vi "Write useUTC.vi"(8 "error in (no error)":errorcluster, 10 "useUTC":bool, 11 "Layout in":refnum<class "Layout.lvclass">) -> (0 "error out":errorcluster, 3 "Layout out":refnum<class "Layout.lvclass">)   [LabVIEW 2026, in "Lumberjack.lvlib" / "Layout.lvclass"]
uses:
  Layout.lvclass
  Layout.lvclass/Layout.ctl
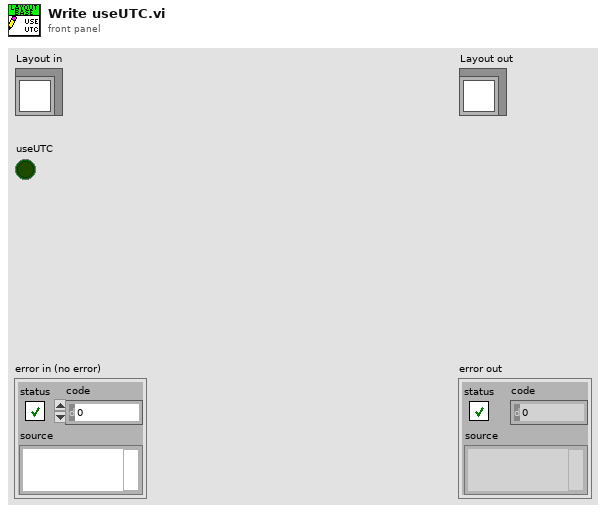
[diagram p1: front panel]
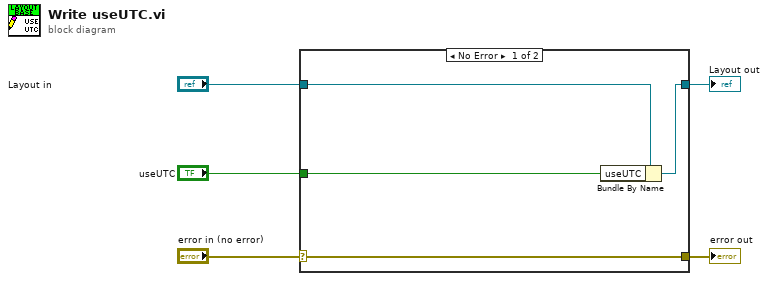
[diagram p0: block diagram]
diagram:
  n1 = case shown="No Error" "error in (no error)" {
    selector: "error in (no error)" -> [w9 w10]
    tunnel: [w9 w10] -> w4
    tunnel: [w7 w11] -> w2
    tunnel: "Layout in" -> [w8 w11]
    tunnel: "useUTC" -> [w6 _]
    frame No Error {
      n2 = Bundle By Name(cluster=w8, "useUTC"=w6) -> (w7:refnum<class "Layout.lvclass">)
    }
    frame Error {
    }
  }
  "error out" <- w4
  "Layout out" <- w2
